vi "Post Substeps Digital Output Task.vi"(9 "DOWrite":T1, 10 "Socket No":u16=1, 11 "Sequence Context In":refnum<k7>) -> (0 "error out":errorcluster, 2 "PhysicalChannel":string[](array[string]), 3 "Report Text":string)   [LabVIEW 2023, in "LTT_TeststandSteptypes.lvlib"]
doc: "This VI Is Socket Number based AO Data Signal Write Through Q"
uses:
  LTT_TeststandSteptypes.lvlib
  HardwareAbstractionLayer_LVOOP/Digital Output/DO_class/DO DAQ/Control/DO Write Enable.ctl
  HardwareAbstractionLayer_LVOOP/Main/Class Options.ctl
  HardwareAbstractionLayer_LVOOP/Digital Output/DO_class/DO.lvclass
  HardwareAbstractionLayer_LVOOP/Main/Main.lvclass
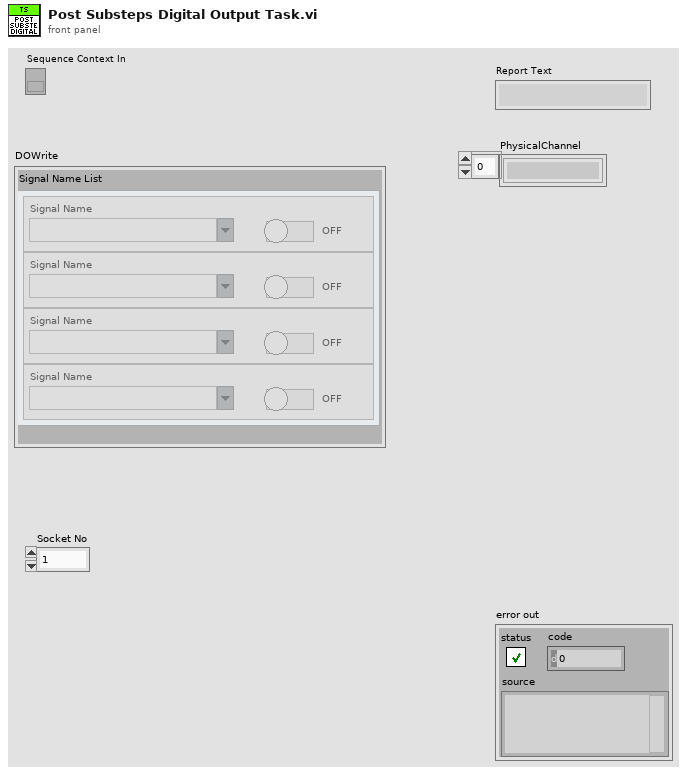
[diagram p1: front panel]
types:
  T1 = typedef "HardwareAbstractionLayer_LVOOP.lvlib/DO.lvclass/DO Write Enable.ctl" = cluster{"Signal Name List":cluster{"Signal Name":string, "Enable Output":bool}[]}
  T2 = typedef "HardwareAbstractionLayer_LVOOP.lvlib/Main.lvclass/Class Options.ctl" = enum16{"Init All Class", "Read All Class", "Write AI Class", "Write AO Class", "Write AO Waveform Generation", "Write DI Class", "Write DO Class", "Write PWM Input Class", "Write PWM Output Class", "Exit"}
  T3 = typedef "HardwareAbstractionLayer_LVOOP.lvlib/Main.lvclass/Class Ref.ctl" = cluster{"FGV":refnum<class "Function Global Variable.lvclass">, "Notifier":refnum<class "NotifierHandler.lvclass">, "Queue":refnum<class "Queue Handler.lvclass">, "User Event":refnum<class "User Event.lvclass">, "Data Manager":refnum<class "Data Manager.lvclass">, "DMM":refnum<class "DMM.lvclass">, "Function Generator":refnum<class "Function Generator.lvclass">, "Oscilloscope":refnum<class "Oscilloscope.lvclass">, "PowerSupply":refnum<class "PowerSupply.lvclass">, "Teststand":refnum<class "Teststand.lvclass">, "AO":refnum<class "AO.lvclass">, "AI":refnum<class "AI.lvclass">, "Database":refnum<class "Database.lvclass">, "AO Waveform Generation":refnum<class "AO.lvclass">, "DO":refnum<class "DO.lvclass">, "DI":refnum<class "DI.lvclass">, "PWM Output":refnum<class "PWM Output.lvclass">, "PWM Input":refnum<class "PWM Input.lvclass">, "RelayOutput":refnum<class "NISwitch.lvclass">, "Modbus":refnum<class "Modbus.lvclass">, "CAN":refnum<class "CAN.lvclass">}
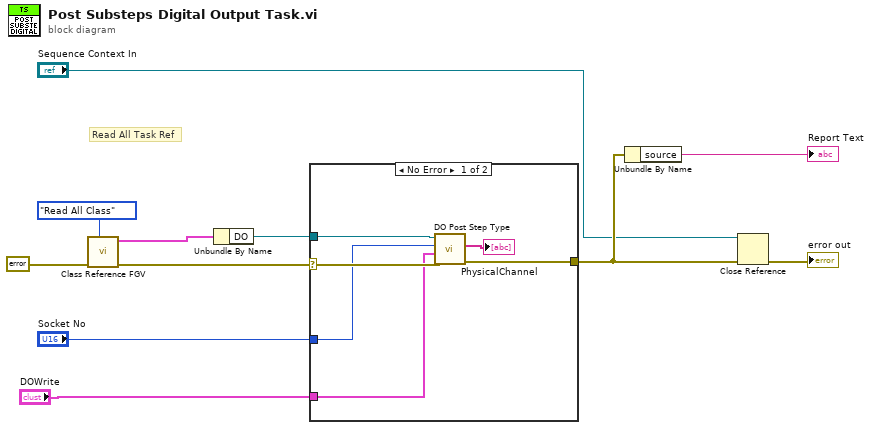
[diagram p0: block diagram]
diagram:
  # "Read All Task Ref"
  n1 = call "Class Reference FGV.vi"("Options"=Class_Options."Read All Class", "error in"=errorcluster {"status"=FALSE, "code"=0, "source"=""}) -> ("error out"=w5:errorcluster, "Class Cluster Out"=w3:T3)  [unwired: 8 in]
  n2 = Unbundle By Name(w3) -> ("DO"=w1:refnum<class "DO.lvclass">)
  n3 = case shown="No Error" w5 {
    selector: w5 -> [w17 w18]
    tunnel: [w16 w18] -> w11
    tunnel: "Socket No" -> [w15 _]
    tunnel: w1 -> [w13 _]
    tunnel: "DOWrite" -> [w14 _]
    frame No Error {
      n4 = call-dynamic "DO Post Step Type.vi"("error in (no error)"=w17, "DOWrite"=w14, "Socket No"=w15, "DO in"=w13) -> ("error out"=w16:errorcluster, "PhysicalChannel"=→"PhysicalChannel":string[])  [unwired: 5 in, 1 out]
    }
    frame Error {
    }
  }
  n5 = Unbundle By Name(w11) -> ("source"=→"Report Text":string)
  n6 = Close Reference(reference="Sequence Context In", error in (no error)=w11) -> (error out=→"error out":errorcluster)
